vi "testInitMission.vi"() -> ()   [LabVIEW 2013]
uses:
  Data/TypeDefs/MissionTypeControl.ctl
  Data/TypeDefs/UTM Location.ctl
  Idle/Idle.lvclass
  GoTo/GoTo.lvclass
  RoundBouy/RoundBouy.lvclass
  PassBouy/PassBouy.lvclass
  StationKeeping/StationKeeping.lvclass
  GenericMission.lvclass
  Waypoint/Waypoint.lvclass
panel:
  in  "Duration (s)":dbl=-1.0
  in  "Tolerance (m)":dbl
  in  "PoI 2":T1 {"North" format="%#_10f"; "East" format="%#_8f"}
  in  "PoI 1":T1 {"North" format="%#_10f"; "East" format="%#_8f"}
  out "Waypoints out":T1[](array[typedef]) {"North" format="%#_10f"; "East" format="%#_8f"}
  in  "Mission Type":T2
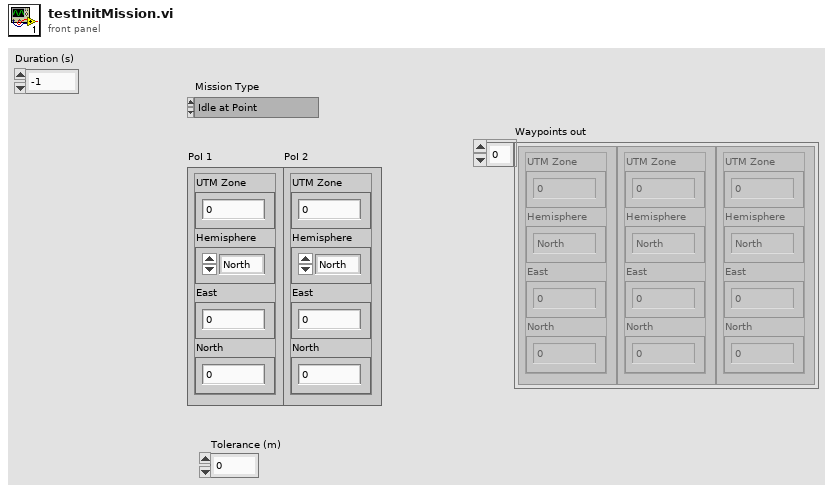
[diagram p1: front panel]
types:
  T1 = typedef "UTM Location.ctl" = cluster{"UTM Zone":dbl, "Hemisphere":enum16{"North", "South"}, "East":dbl, "North":dbl}
  T2 = typedef "MissionTypeControl.ctl" = enum16{"Idle at Point", "Drive to Waypoint", "Round Buoy to Port", "Round Buoy to Starboard", "Pass Between Buoys", "Station Keeping"}
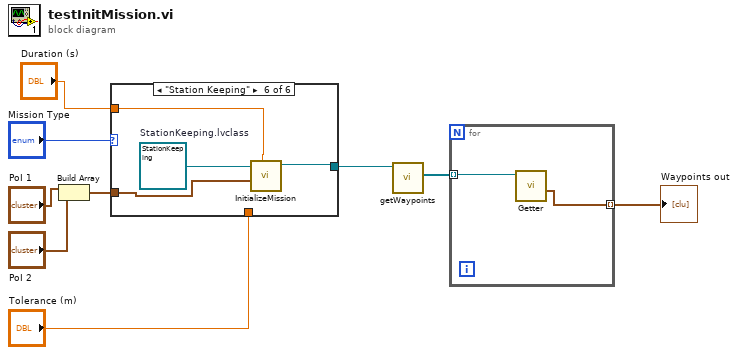
[diagram p0: block diagram]
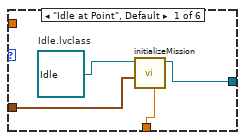
[diagram p2: hidden frame]
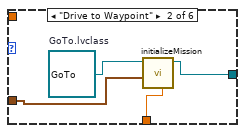
[diagram p3: hidden frame]
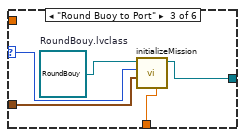
[diagram p4: hidden frame]
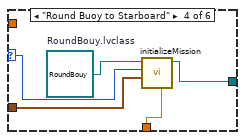
[diagram p5: hidden frame]
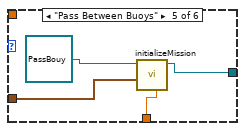
[diagram p6: hidden frame]
diagram:
  n1 = Build Array("PoI 1", "PoI 2") -> (w4:T1[])
  n2 = case shown="\"Station Keeping\"" "Mission Type" {
    selector: "Mission Type" -> [_ _ w21 w26 _ _]
    tunnel: w4 -> [w12 w16 w20 w25 w30 w34]
    tunnel: "Tolerance (m)" -> [w10 w15 w19 w24 w31 _]
    tunnel: [w11 w14 w18 w23 w29 w32] -> w2
    tunnel: "Duration (s)" -> [_ _ _ _ _ w33]
    frame "Idle at Point", Default {
      w13 = refnum<class "Idle.lvclass"> refnum  # Idle.lvclass
      n3 = call-dynamic "initializeMission.vi"("Tolerance (m)"=w10, "Points of Interest"=w12, "Idle in"=w13) -> ("Idle out"=w11:refnum<class "Idle.lvclass">)  [unwired: 7 in, 1 out]
    }
    frame "Drive to Waypoint" {
      w17 = refnum<class "GoTo.lvclass"> refnum  # GoTo.lvclass
      n4 = call-dynamic "initializeMission.vi"("Tolerance (m)"=w15, "Points of Interest"=w16, "GoTo in"=w17) -> ("GoTo out"=w14:refnum<class "GoTo.lvclass">)  [unwired: 7 in, 1 out]
    }
    frame "Round Buoy to Port" {
      w22 = refnum<class "RoundBouy.lvclass"> refnum  # RoundBouy.lvclass
      n5 = call-dynamic "initializeMission.vi"("Tolerance (m)"=w19, "Points of Interest"=w20, "Mission Type"=w21, "RoundBouy in"=w22) -> ("RoundBouy out"=w18:refnum<class "RoundBouy.lvclass">)  [unwired: 6 in, 1 out]
    }
    frame "Round Buoy to Starboard" {
      w27 = refnum<class "RoundBouy.lvclass"> refnum  # RoundBouy.lvclass
      n6 = call-dynamic "initializeMission.vi"("Tolerance (m)"=w24, "Points of Interest"=w25, "Mission Type"=w26, "RoundBouy in"=w27) -> ("RoundBouy out"=w23:refnum<class "RoundBouy.lvclass">)  [unwired: 6 in, 1 out]
    }
    frame "Pass Between Buoys" {
      n7 = call-dynamic "initializeMission.vi"("Tolerance (m)"=w31, "Points of Interest"=w30, "PassBouy.lvclass"=refnum<class "PassBouy.lvclass"> refnum) -> ("PassBouy.lvclass out"=w29:refnum<class "PassBouy.lvclass">)  [unwired: 7 in, 1 out]
    }
    frame "Station Keeping" {
      w35 = refnum<class "StationKeeping.lvclass"> refnum  # StationKeeping.lvclass
      n8 = call-dynamic "InitializeMission.vi"("Duration (s)"=w33, "Points of Interest"=w34, "StationKeeping in"=w35) -> ("StationKeeping out"=w32:refnum<class "StationKeeping.lvclass">)  [unwired: 7 in, 1 out]
    }
  }
  n9 = call-dynamic "getWaypoints.vi"("GenericMission in"=w2) -> ("Waypoint Array"=w8:refnum<class "Waypoint.lvclass">[])  [unwired: 8 in, 2 out]
  n10 = for {
    tunnel: w8 -> [w37] mode=indexing
    tunnel: [w36] -> w7 mode=indexing
    n11 = call "Getter.vi"("Waypoint In"=w37) -> ("Coords"=w36:T1)  [unwired: 6 in, 4 out]
  }
  "Waypoints out" <- w7
